vi "GetDeviceFirmwareInfo.vi"(8 "timeout (10000)":i32=2000, 10 "IP":string="10.2.104.72") -> (1 "ConnectedToWebService":bool, 3 "AppVersion":T1)   [LabVIEW 2017]
uses:
  <vilib>/httpClient/LabVIEWHTTPClient.lvlib
panel:
  out "resulting string":string
  out "error out":errorcluster
  out "body":string
  in  "Port":u16=8002 step=1
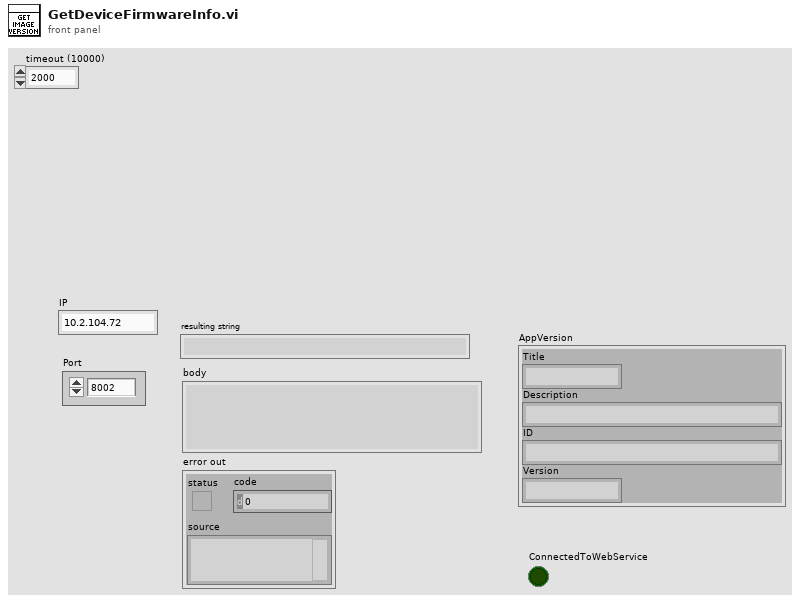
[diagram p1: front panel]
types:
  T1 = cluster{"Title":string, "Description":string, "ID":string, "Version":string}
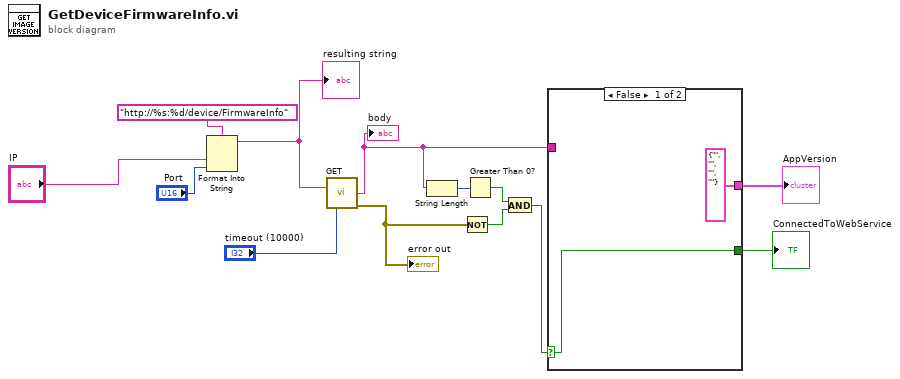
[diagram p0: block diagram]
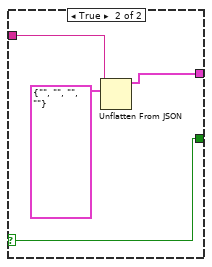
[diagram p2: hidden frame]
diagram:
  n1 = Format Into String(format string="http://%s:%d/device/FirmwareInfo", "IP", "Port") -> (resulting string=w11:string)  [unwired: 2 in, 1 out]
  "resulting string" <- w11
  n2 = call <vilib>:"GET.vi"("url"=w11, "timeout (10000)"="timeout (10000)") -> ("body"=w9:string, "error out"=w7:errorcluster)  [unwired: 10 in, 2 out]
  "body" <- w9
  "error out" <- w7
  n3 = String Length(string=w9) -> (length=w8:i32)
  n4 = Not(x=w7) -> (.not. x?=w4:bool)
  n5 = Greater Than 0?(x=w8) -> (x > 0?=w5:bool)
  n6 = And(x=w5, y=w4) -> (x .and. y?=w6:bool)
  n7 = case shown="False" w6 {
    selector: w6 -> [w15 w17]
    tunnel: w9 -> [_ w19]
    tunnel: [w15 w17] -> w3
    tunnel: [T1 {"Title"="", "Description"="", "ID"="", "Version"=""} w16] -> w2
    frame False {
    }
    frame True {
      n8 = Unflatten From JSON(JSON string=w19, type and defaults=T1 {"Title"="", "Description"="", "ID"="", "Version"=""}) -> (value=w16:T1)  [unwired: 5 in, 1 out]
    }
  }
  "ConnectedToWebService" <- w3
  "AppVersion" <- w2
